vi "P2.vi"() -> ()   [LabVIEW 2013]
uses:
  <vilib>/measure/NI_MABase.lvlib
  <vilib>/measure/NI_MAPro.lvlib
  <vilib>/measure/macond.llb/Continuous Waveform Convolution for 1 Chan.vi
  <vilib>/Analysis/NI_AALBase.lvlib
panel:
  out "Waveform Graph":dbl[](graph)
  in  "FRECUENCIA":dbl
  in  "NIVEL DE RUIDO":dbl
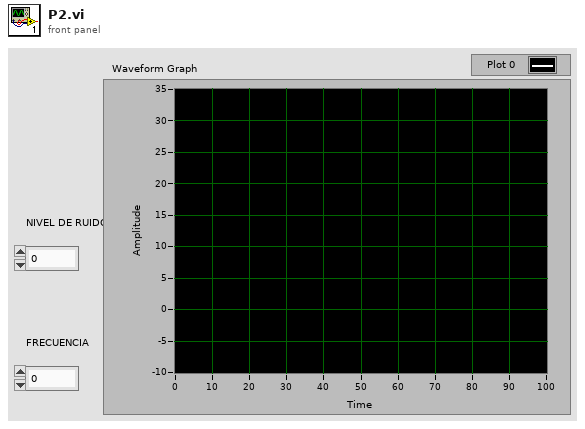
[diagram p1: front panel]
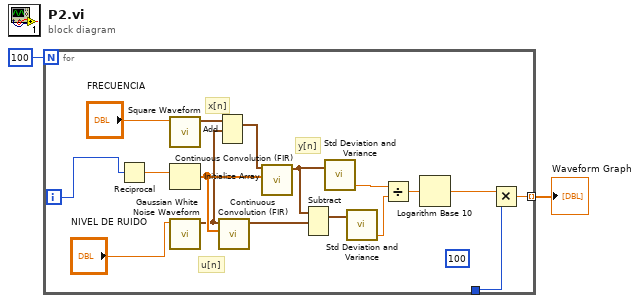
[diagram p0: block diagram]
diagram:
  n1 = for {
    N: 100 -> [_]
    tunnel: [w8] -> w2 mode=indexing
    tunnel: _ -> [w7]
    i -> [w3]
    w4 = 100
    # "y[n]"
    # "u[n]"
    # "x[n]"
    n2 = Reciprocal(x=w3) -> (1/x=w16:dbl)
    n3 = call <vilib>:"Square Waveform.vi"("frequency"="FRECUENCIA") -> ("signal out"=w18:waveform(dbl))  [unwired: 9 in, 1 out]
    n4 = Initialize Array(w16) -> (w15:dbl[])  [unwired: 1 in]
    n5 = call <vilib>:"Gaussian White Noise Waveform.vi"("standard deviation"="NIVEL DE RUIDO") -> ("signal out"=w5:waveform(dbl))  [unwired: 9 in, 1 out]
    n6 = Add(1:w5, 2:w18) -> (0:w17:waveform(dbl))  [unwired: 1 in, 1 out]
    n7 = call-poly <vilib>:"Continuous Convolution (FIR).vi"("kernel"=w15, "signal in"=w5) -> ("signal out"=w6:waveform(dbl))  [unwired: 8 in, 1 out]
    n8 = call-poly <vilib>:"Continuous Convolution (FIR).vi"("kernel"=w15, "signal in"=w17) -> ("signal out"=w13:waveform(dbl))  [unwired: 8 in, 1 out]
    n9 = Subtract(1:w6, 2:w13) -> (0:w14:waveform(dbl))  [unwired: 1 in, 1 out]
    n10 = call <vilib>:"Std Deviation and Variance.vi"("X"=w13) -> ("variance"=w11:dbl)  [unwired: 1 in, 2 out]
    n11 = call <vilib>:"Std Deviation and Variance.vi"("X"=w14) -> ("variance"=w10:dbl)  [unwired: 1 in, 2 out]
    n12 = Divide(x=w11, y=w10) -> (x/y=w12:dbl)
    n13 = Logarithm Base 10(1:w12) -> (0:w9:dbl)
    n14 = Multiply(x=w9, y=w7) -> (x*y=w8:dbl)
  }
  "Waveform Graph" <- w2
